vi "Timer.vi"(9 "Timer Action (Check)":T1, 10 "Auto Reset? (T)":bool=TRUE, 11 "Timeout (ms)":u32=60000) -> (1 "Elapsed Time (ms)":u32, 3 "Time Elapsed?":bool)   [LabVIEW 2011]
doc: "Resettable Timer VI\n\n<b>Timeout (ms)</b> The length of time for the timer to mark.\n\n<b>Timer Action (Check)</b> The action to take:\n<b>Check</b>\n<b>Start</b>\n<b>Pause</b>\n<b>Resume</b>\n<b>Stop</b>\n\n<b>Time Elapsed?</b> Indicator of whether the time has elapsed.\n<b>Elapsed Time (ms)</b> Time in milliseconds that have elapsed thus far.\n\n\nVersion 1.0 - 10/21/2009\n\nPhaeron, Inc.\nwww.phaeron.com\ninfo@phaeron.com"
uses:
  TimerAction.ctl
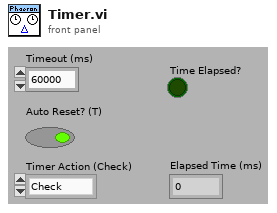
[diagram p1: front panel]
types:
  T1 = typedef "TimerAction.ctl" = enum16{"Check", "Start", "Pause", "Resume", "Stop", "Restart", "Init All"}
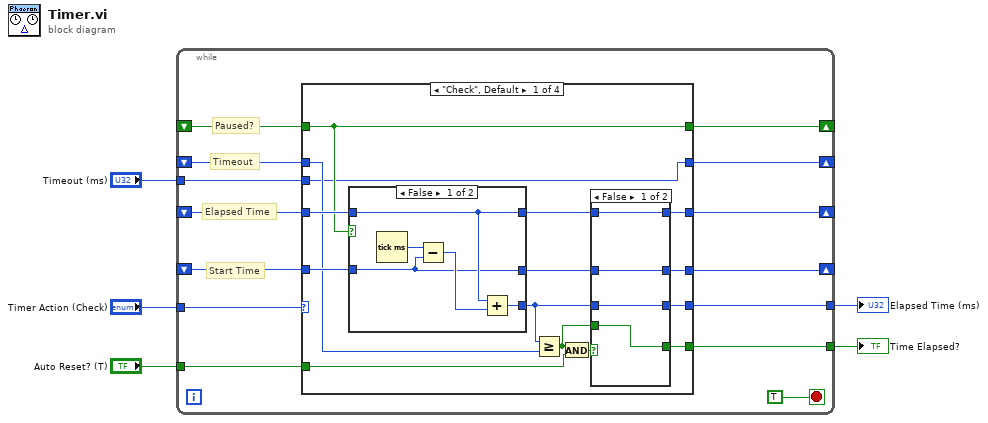
[diagram p0: block diagram]
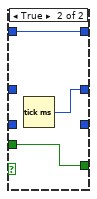
[diagram p2: hidden frame]
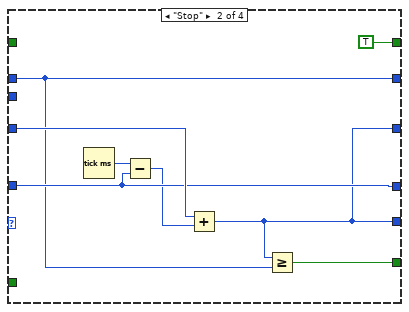
[diagram p4: hidden frame]
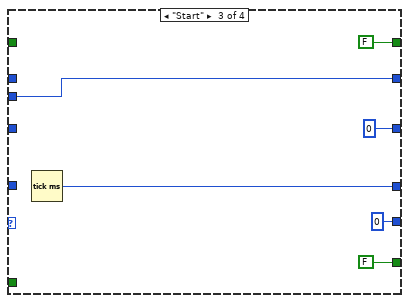
[diagram p5: hidden frame]
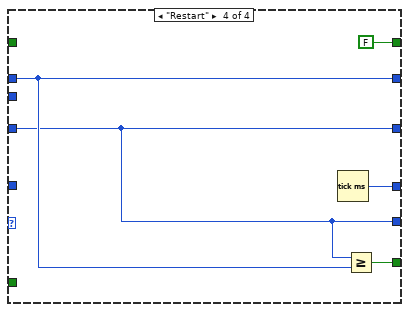
[diagram p6: hidden frame]
diagram:
  n1 = while {
    tunnel: "Timer Action (Check)" -> [w18]
    tunnel: "Timeout (ms)" -> [w17]
    shift-right: [w16] -> _
    shift-left: _ -> [w15]
    shift-right: [w14] -> _
    shift-left: _ -> [w13]
    shift-right: [w12] -> _
    shift-left: _ -> [w11]
    tunnel: [w10] -> w3
    tunnel: [w9] -> w2
    shift-right: [w8] -> _
    shift-left: _ -> [w7]
    tunnel: "Auto Reset? (T)" -> [w6]
    stop <- TRUE stop-if-true
    # "Paused?"
    # "Elapsed Time"
    # "Start Time"
    # "Timeout"
    n2 = case shown="\"Check\", Default" w18 {
      tunnel: w17 -> [w23 _ w62 _]
      tunnel: [w23 w52 w62 w66] -> w16
      tunnel: w15 -> [w26 w52 _ w66]
      tunnel: [w30 w54 w61 w65] -> w14
      tunnel: w13 -> [w33 w54 _ _]
      tunnel: [w24 w49 u32 0 w64] -> w12
      tunnel: w11 -> [w34 w56 _ w64]
      tunnel: [w28 w49 u32 0 w64] -> w10
      tunnel: [w29 w51 FALSE w67] -> w9
      tunnel: [w32 TRUE FALSE FALSE] -> w8
      tunnel: w7 -> [w32 _ _ _]
      tunnel: w6 -> [w21 _ _ _]
      frame "Check", Default {
        n3 = case shown="False" w32 {
          tunnel: w34 -> [w43 w47]
          tunnel: w33 -> [w42 w48]
          tunnel: [w44 w47] -> w27
          tunnel: [w43 w47] -> w25
          tunnel: [w42 w48] -> w31
          frame False {
            n4 = Tick Count (ms)() -> (millisecond timer value=w46:u32)
            n5 = Subtract(x=w46, y=w42) -> (x-y=w45:u32)
            n6 = Add(x=w43, y=w45) -> (x+y=w44:u32)
          }
          frame True {
          }
        }
        n7 = Greater Or Equal?(x=w27, y=w26) -> (x >= y?=w20:bool)
        n8 = And(x=w20, y=w21) -> (x .and. y?=w22:bool)
        n9 = case shown="False" w22 {
          tunnel: w31 -> [w37 _]
          tunnel: [w37 w41] -> w30
          tunnel: [w35 w39] -> w29
          tunnel: [w38 _] -> w28
          tunnel: w27 -> [w38 _]
          tunnel: w25 -> [w36 w40]
          tunnel: [w36 w40] -> w24
          tunnel: w20 -> [w35 w39]
          frame False {
          }
          frame True {
            n10 = Tick Count (ms)() -> (millisecond timer value=w41:u32)
          }
        }
      }
      frame "Stop" {
        n11 = Tick Count (ms)() -> (millisecond timer value=w55:u32)
        n12 = Subtract(x=w55, y=w54) -> (x-y=w53:u32)
        n13 = Add(x=w56, y=w53) -> (x+y=w49:u32)
        n14 = Greater Or Equal?(x=w49, y=w52) -> (x >= y?=w51:bool)
      }
      frame "Start" {
        n15 = Tick Count (ms)() -> (millisecond timer value=w61:u32)
      }
      frame "Restart" {
        n16 = Tick Count (ms)() -> (millisecond timer value=w65:u32)
        n17 = Greater Or Equal?(x=w64, y=w66) -> (x >= y?=w67:bool)
      }
    }
  }
  "Elapsed Time (ms)" <- w3
  "Time Elapsed?" <- w2
